vi "NeuralNetwork.vi"() -> ()   [LabVIEW 2014]
panel:
  out "output":dbl[](array[numeric])
  in  "Enum":enum16{"X", "Y", "Z"}(ring)
  in  "stop":bool
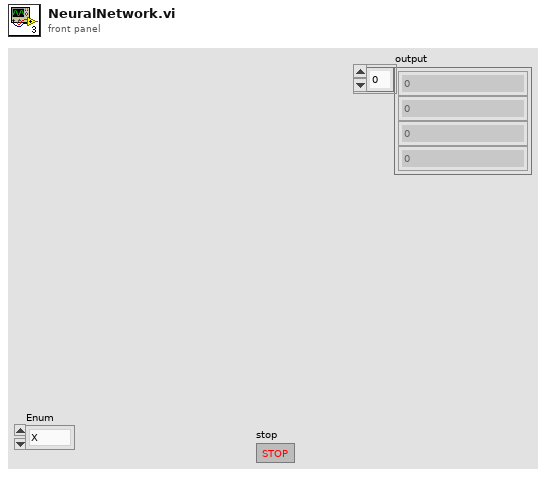
[diagram p1: front panel]
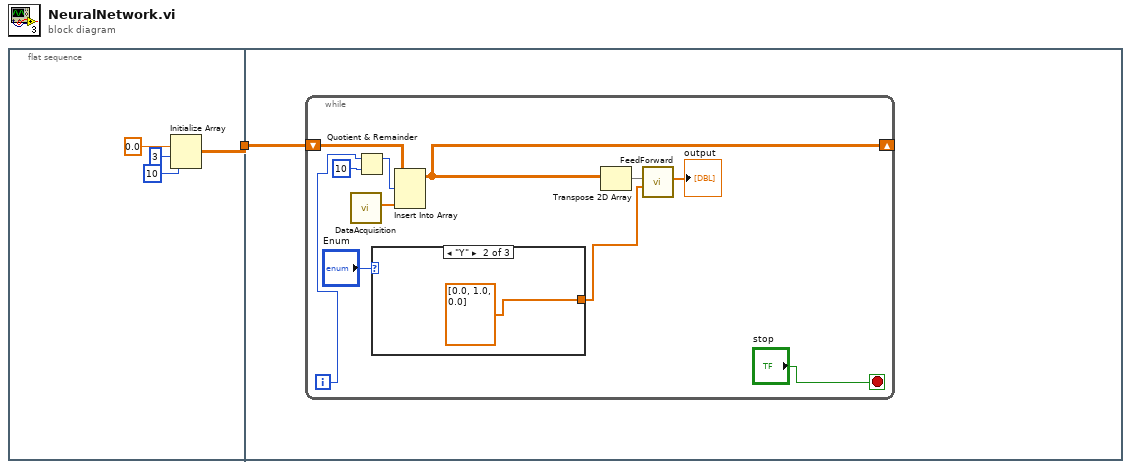
[diagram p0: block diagram]
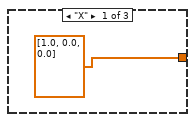
[diagram p2: hidden frame]
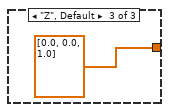
[diagram p3: hidden frame]
diagram:
  n1 = flat-sequence {
    tunnel: [w5] -> w1
    tunnel: w1 -> [w6]
    frame #0 {
      n2 = Initialize Array(0.0, 3 ("dimension size"), 10 ("dimension size")) -> (w5:dbl[][])
    }
    frame #1 {
      n3 = while {
        shift-right: [w7] -> _
        shift-left: w6 -> [w13]
        i -> [w12]
        stop <- "stop" stop-if-true
        n4 = call "DataAcquisition.vi"() -> ("appended array"=w9:dbl[])  [unwired: 10 in, 1 out]
        n5 = Quotient & Remainder(x=w12, y=10) -> (x-y*floor(x/y)=w10:i32)  [unwired: 1 out]
        n6 = case shown="\"Y\"" "Enum" {
          tunnel: [dbl[] [1.0, 0.0, 0.0] ("opinons") dbl[] [0.0, 1.0, 0.0] ("opinons") dbl[] [0.0, 0.0, 1.0] ("opinons")] -> w16
          frame "X" {
          }
          frame "Y" {
          }
          frame "Z", Default {
          }
        }
        n7 = Insert Into Array(array=w13, index (row)=w10, new element=w9) -> (w7:dbl[][])  [unwired: 1 in]
        n8 = Transpose 2D Array(2D array=w7) -> (transposed array=w8:dbl[][])
        n9 = call "FeedForward.vi"("opinons"=w16, "inputs"=w8) -> ("output"=→"output":dbl[])  [unwired: 9 in]
      }
    }
  }
